vi "queue-cleanup.vi"(11 "Queue in":refnum<queue>) -> (3 "queue name":string)   [LabVIEW 2013]
uses:
  bp_work_unit.ctl
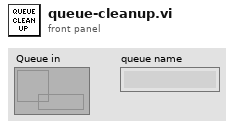
[diagram p1: front panel]
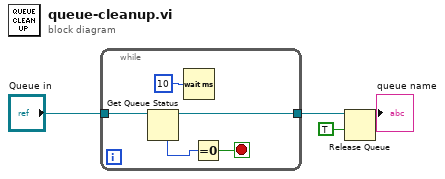
[diagram p0: block diagram]
diagram:
  n1 = while {
    tunnel: [w7] -> w1
    tunnel: "Queue in" -> [w5]
    stop <- w8 stop-if-true
    n2 = Get Queue Status(queue=w5) -> (queue out=w7:refnum<queue>, # elements in queue=w9:i32)  [unwired: 2 in, 6 out]
    n3 = Wait (ms)(milliseconds to wait=u32 10) -> ()  [unwired: 1 out]
    n4 = Equal To 0?(x=w9) -> (x = 0?=w8:bool)
  }
  n5 = Release Queue(queue=w1, force destroy? (F)=TRUE) -> (queue name=→"queue name":string)  [unwired: 1 in, 2 out]
